vi "Ranked Integrated Correlation 2D.vi"(6 "Radius (cm)":dbl=123.4 format="%#_13g", 9 "Sampling Rate":i32=500000, 11 "Waveforms":waveform(dbl)[](array[waveform])) -> (2 "Source Coordinates (cm, cm)":cluster{"x":dbl, "y":dbl})   [LabVIEW 2013]
uses:
  <vilib>/Waveform/WDTOps.llb/WDT Index Channel DBL.vi
  <vilib>/Analysis/2dsp.llb/1D Cross Correlation (DBL).vi
  <vilib>/Analysis/NI_AALPro.lvlib
panel:
  out "Ranked Delays":dbl[](array[numeric])
  out "Ranked (Row, Column)":dbl[][](array[numeric])
  out "Row":i32
  out "Page":i32
  out "Rxy 2":dbl[][][](array[numeric])
  out "Cross Corr.\n1/2 Length":i32
  out "Signals":waveform(dbl)[](graph)
  out "Correlation":dbl[](graph)
  out "Lag Matrix":dbl[][](array[numeric])
  # "Inputs and Outputs"
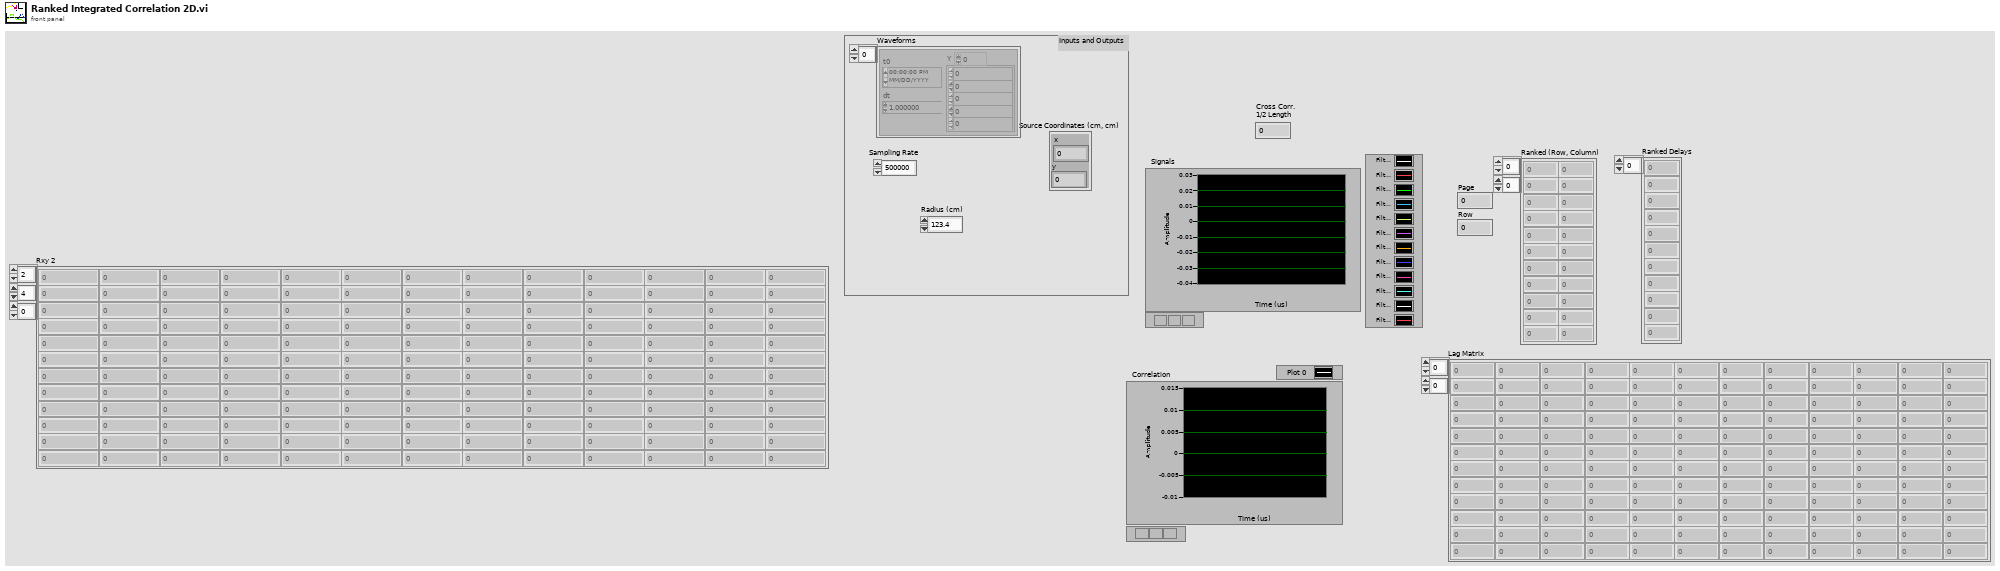
[diagram p1: front panel]
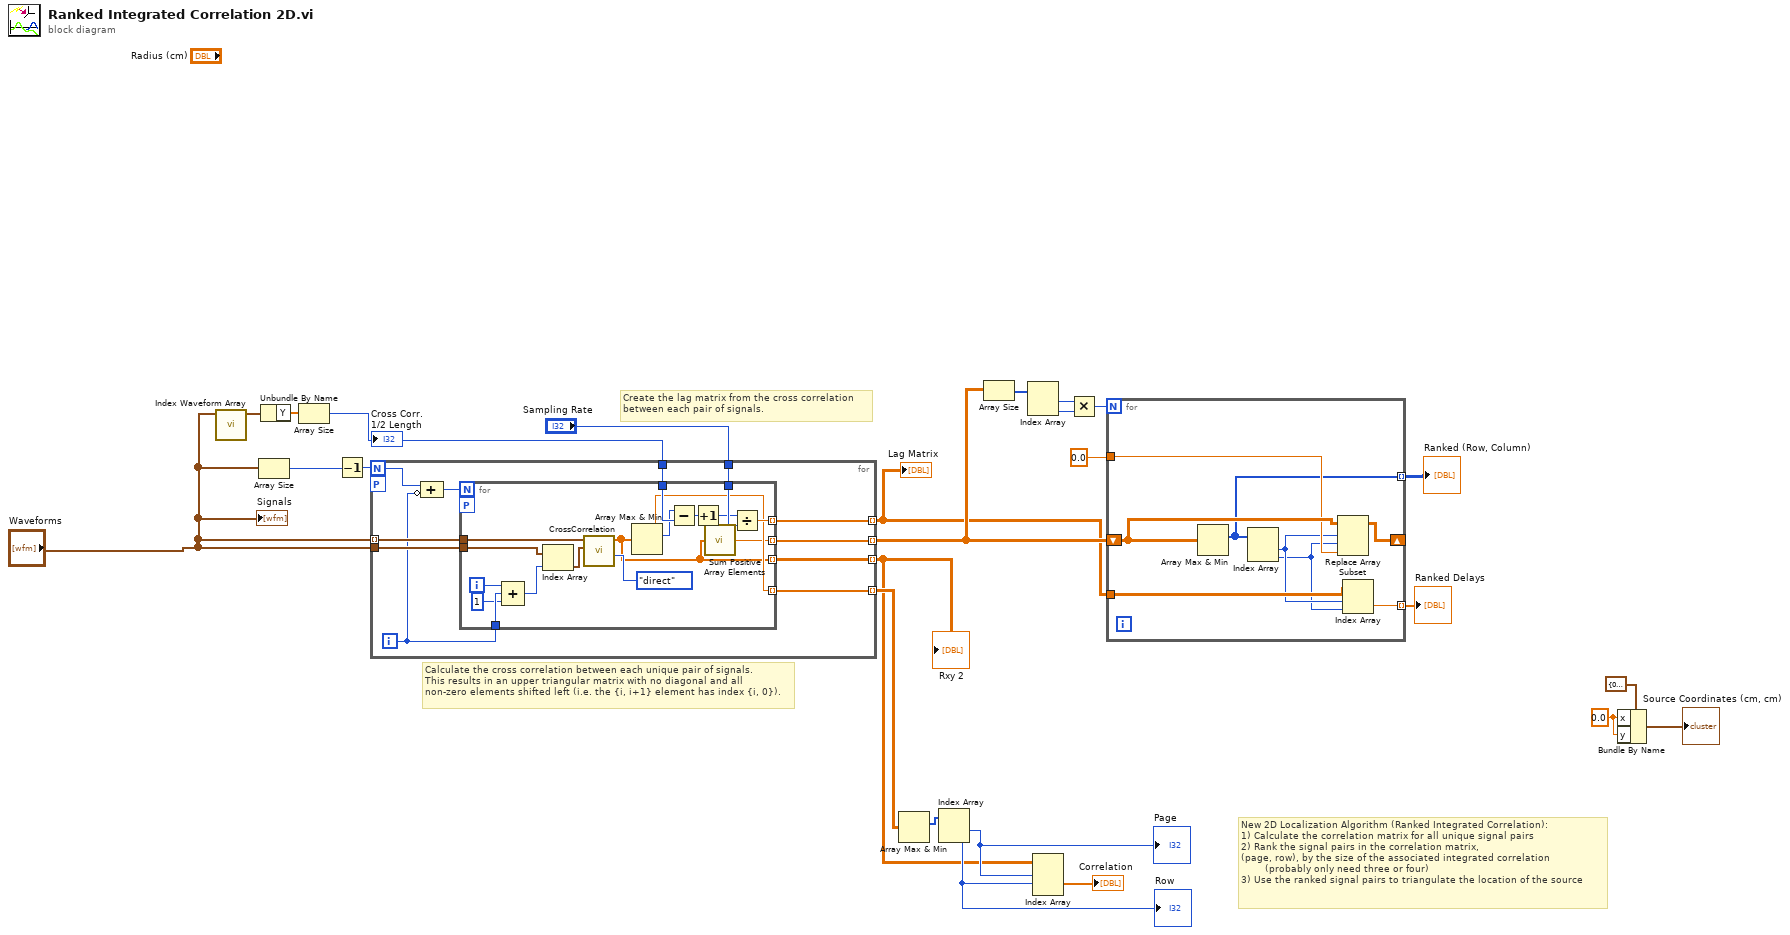
[diagram p0: block diagram]
diagram:
  w4 = 0.0 ("x")
  # "New 2D Localization Algorithm (Ranked Integrated Correlation):\n1) Calculate the correlation matrix for all unique signal pairs\n2) Rank the signal pairs in the correlation matrix,\n(page, row), by the size of the associated integrated correlation\n        (probably only need three or four)\n3) Use the ranked signal pairs to triangulate the location of the source"
  # "Calculate the cross correlation between each unique pair of signals.\nThis results in an upper triangular matrix with no diagonal and all\nnon-zero elements shifted left (i.e. the {i, i+1} element has index {i, 0})."
  # "Create the lag matrix from the cross correlation\nbetween each pair of signals."
  n1 = call-poly <vilib>:"Index Waveform Array.vi"("waveform array"="Waveforms") -> ("waveform"=w19:waveform(dbl))  [unwired: 9 in, 1 out]
  n2 = Array Size ("Size(s)")(array="Waveforms") -> (size(s)=w21:i32)
  n3 = Unbundle By Name(w19) -> ("Y"=w18:dbl[])
  n4 = Array Size(array=w18) -> (size(s)=w17:i32)
  "Cross Corr.\n1/2 Length" <- w17
  n5 = Decrement(x=w21) -> (x-1=w22:i32)
  n6 = for {
    N: w22 -> [w29]
    tunnel: "Waveforms" -> [w32] mode=indexing
    tunnel: "Waveforms" -> [w36]
    tunnel: "Sampling Rate" -> [w35]
    tunnel: [w34] -> w2 mode=indexing
    tunnel: [w33] -> w7 mode=indexing
    tunnel: w17 -> [w31]
    workers-P: _ -> [_]
    tunnel: [w27] -> w16 mode=indexing
    tunnel: [w26] -> w6 mode=indexing
    i -> [w28]
    n7 = Compound Arithmetic op=ADD(w29, invert w28) -> (w30:i32)
    n8 = for {
      N: w30 -> [_]
      tunnel: w36 -> [w43]
      tunnel: w32 -> [w53]
      tunnel: w35 -> [w52]
      tunnel: [w51] -> w34 mode=indexing
      tunnel: [w38] -> w33 mode=indexing
      tunnel: w31 -> [w48]
      tunnel: w28 -> [w45]
      workers-P: _ -> [_]
      tunnel: [w40] -> w27 mode=indexing
      tunnel: [w37] -> w26 mode=indexing
      i -> [w46]
      n9 = Compound Arithmetic op=ADD(w46, w45, 1 ("value")) -> (w44:i32)
      n10 = Index Array(array=w43, index=w44) -> (element=w42:waveform(dbl))
      n11 = call-poly <vilib>:"CrossCorrelation.vi"("algorithm"=enum32{"direct", "frequency domain"}."direct", "Y"=w42, "X"=w53) -> ("Rxy"=w38:dbl[])  [unwired: 7 in, 1 out]
      n12 = Array Max & Min(array=w38) -> (max value=w40:dbl, max index (indices)=w39:i32)  [unwired: 2 out]
      n13 = Subtract(x=w39, y=w48) -> (x-y=w50:i32)
      n14 = Increment(x=w50) -> (x+1=w49:i32)
      n15 = call "Sum Positive Array Elements.vi"("Array"=w38) -> ("Positive Element Sum"=w37:dbl)  [unwired: 4 in]
      n16 = Divide(x=w49, y=w52) -> (x/y=w51:dbl)
    }
  }
  "Lag Matrix" <- w2
  "Rxy 2" <- w7
  n17 = Array Max & Min(array=w16) -> (max index (indices)=w15:i32[])  [unwired: 3 out]
  n18 = Index Array(array=w15) -> (element #1=w14:i32, element #2=w13:i32)  [unwired: 2 in]
  "Page" <- w14
  "Row" <- w13
  n19 = Array Size(array=w6) -> (size(s)=w11:i32[])
  n20 = Index Array(array=w11) -> (element #1=w9:i32, element #2=w10:i32)  [unwired: 2 in]
  n21 = Index Array(array=w7, index (dim 0)=w14, index (dim 1)=w13) -> (element=→"Correlation":dbl[])  [unwired: 1 in]
  n22 = Multiply(x=w9, y=w10) -> (x*y=w8:i32)
  n23 = for {
    N: w8 -> [_]
    shift-right: [w58] -> _
    shift-left: w6 -> [w61]
    tunnel: 0.0 ("element") -> [w60]
    tunnel: [w59] -> w3 mode=indexing
    tunnel: w2 -> [w57]
    tunnel: [w54] -> w1 mode=indexing
    n24 = Array Max & Min(array=w61) -> (max index (indices)=w59:i32[])  [unwired: 3 out]
    n25 = Index Array(array=w59) -> (element #1=w56:i32, element #2=w55:i32)  [unwired: 2 in]
    n26 = Replace Array Subset(array=w61, new element=w60, index (row)=w56, index (col)=w55) -> (w58:dbl[][])
    n27 = Index Array(array=w57, index (row)=w56, index (col)=w55) -> (element=w54:dbl)
  }
  "Ranked (Row, Column)" <- w3
  "Ranked Delays" <- w1
  n28 = Bundle By Name(cluster=cluster{"x":dbl, "y":dbl} {"x"=0.0, "y"=0.0} ("Polar\nCoordinates"), "x"=w4, "y"=w4) -> (→"Source Coordinates (cm, cm)":cluster{"x":dbl, "y":dbl})
  "Signals" <- "Waveforms"
